vi "AnalysisTools.vi"(7 "Cali.Ref(Caller)":refnum<vi>) -> ()   [LabVIEW 2013]
uses:
  ProcessMethods/Binning/BinType.ctl
  <vilib>/Utility/miscctls.llb/LVRowAndColumnUnsignedTypeDef.ctl
  Files/Signal_Segment.ctl
  ControlDef/ProcessingMode.ctl
  <vilib>/Analysis/6fits.llb/General Linear Fit Algorithm.ctl
  <vilib>/Analysis/6fits.llb/Curve Fitting Criteria.ctl
  UI/Autoscale_Y_Multiple.vi
  ProcessMethods/Binning/SpectraBinning.vi
  ProcessMethods/MassResolutionCalc/FindMassResolution_Multiple.vi
  <vilib>/regexp/Match Regular Expression.xnode
  <vilib>/Analysis/NI_AALPro.lvlib
  <vilib>/Analysis/NI_AAL_SigProc.lvlib
  <vilib>/ptbypt/NI_PtbyPt.lvlib
panel:
  in  "Fullscale Y":bool
  in  "Y--":bool
  in  "Y++":bool
  in  "Res.":bool
  in  "Binning":bool
  in  "BinType":T1
  in  "BinWidth":dbl=1.0 min=0.001 max=32768.0 step=0.001 format="%.3f"
  in  "X++":bool
  in  "X--":bool
  in  "Fullscale X":bool
  in  "Reload":bool
  in  "Path":path
  out "Spectrum":cluster{dbl[], "Amplitudes":dbl[]}[](graph)
  in  "Tab Control":T2(tab)
  in  "Calibration Table":dbl[][](array[numeric]) caption="raw m/z"
  in  "Export_GraphData":bool
  in  "ApplyToFile":bool
  out "M/z curve fitting":cluster{"Y":dbl[], "Y":dbl[]}[](graph)
  in  "Calibration Coefficients":dbl[](array[numeric]) format="%.5f"
  out "R^2":dbl
  in  "Apply":bool
  in  "mzML Export":bool
  in  "ApplyToMainProgram":bool
  in  "AddSelection":bool
  in  "ExportPCA":bool
  in  "Multicolumn Listbox":i32[](listbox)
  in  "Search":bool
  in  "threshold":dbl format="%#_5p"
  in  "width":i32=3 min=3
  out "# found":i32
  in  "LoadMultiple...":bool
  in  "Reset":bool
  in  "ExportTable":bool
  in  "CopyPeakAreas":bool
  in  "CalcPeakAreas":bool
  in  "Selected Peak list":i32[](listbox)=[2]
  in  "Decode_regexp":string="Br2-Tyr_([-+]?[0-9]*[,\\.]?[0-9]+([eE][-+]?[0-9]+)?)%_([-+]?[0-9]*[,\\.]?[0-9]+([eE][-+]?[0-9]+)?)uJ_([-+]?[0-9]*[,\\.]?[0-9]+([eE][-+]?[0-9]+)?)us_([-+]?[0-9]*[,\\.]?[0-9]+([eE][-+]?[0-9]+)?).txt"
  in  "Decode_Filename?":bool
  in  "Accumulate":bool
  out "Accumulated Data":dbl[][](array[numeric])
  in  "Export+Proc":bool
  out "selected submatch":string
  in  "Submatch Selector":i32
  out "Referance Mass":string[][](table)=[["Compound", "", "mass", ""], ["Sexithiophone", "6T", "493.98", "s"], ["", "4T", "330.00", "s"], ["", "8T", "657.96", "w"], ["NPM", "M+", "297", "s"], ["", "", "217", "w"], ["CHCA", "M+", "189.04", "s"], ["DHB", "M+", "154.03", "s"], ["Rifampcin", "", "", ""], ["Tantalum", "", "", ""], ["Cu", "63", "", ""], ["", "65", "", ""], ["Mo", "", "", ""]]
  in  "m/z":dbl
  in  "time":dbl
  in  "Add to":bool
  out "Original m/z":dbl
  in  "Calc Calibration":bool
  in  "Quit":bool
  # "raw m/z"
  # "time"
  # "cali. m/z"
  # "delta m/z"
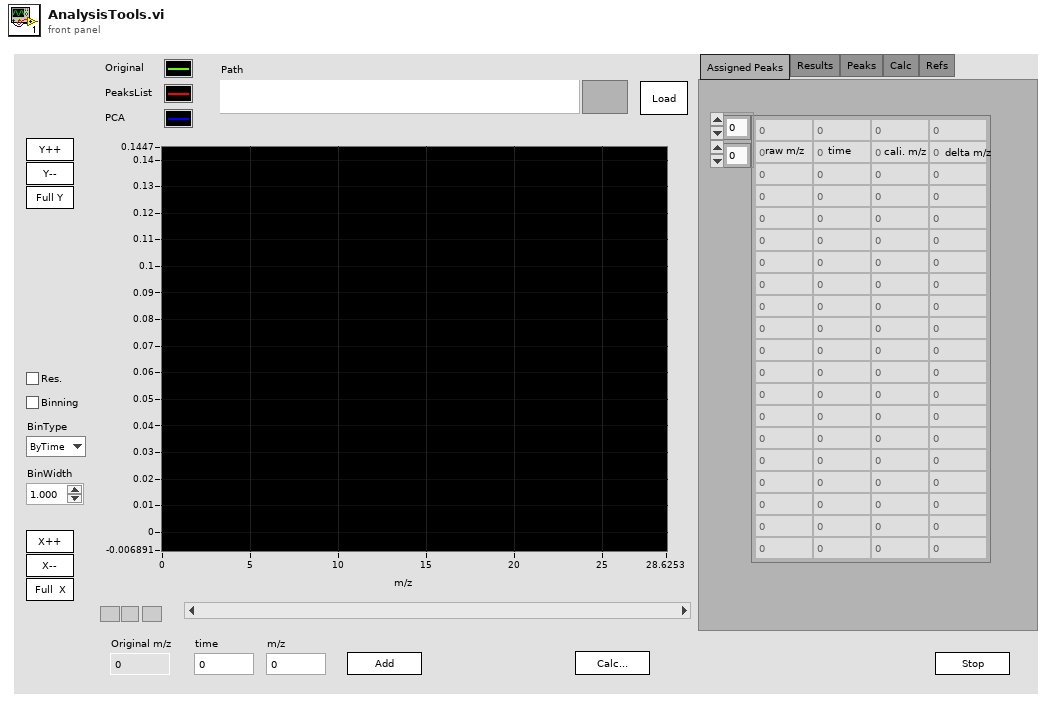
[diagram p1: front panel]
types:
  T1 = typedef "BinType.ctl" = enum16{"ByTime", "ByScreen", "ByMass", "ToUnitMass"}
  T2 = enum32{"Assigned Peaks", "Results", "Peaks", "Calc", "Refs"}
  T3 = typedef "LVRowAndColumnUnsignedTypeDef.ctl" = cluster{"Row":u32, "Column":u32}
  T4 = cluster{"Plot.Bar Plot Style":u8, "Plot.Plot Color":u32, "Plot.Line Style":u8, "Plot.Plot Interpolation":u8, "Plot.Plot Name":string, "Plot.Point Style":u8, "Plot.Visible":bool}[]
  T5 = typedef "Signal_Segment.ctl" = cluster{"SampleRate":dbl, "TrigDelay":dbl, "SpecLength":dbl, "DAQ_Range":dbl, "Average#":i32, "Position":dbl[], "Spectrum":sgl[], "Calibr.":dbl[], "Pressure":dbl, "Desp_LaserEnergy":dbl, "PI_LaserEnergy":dbl, "Voltages Table":sgl[][], "ProcMode":T6, "Threshold":dbl, "Comment":string, "TickCount":dbl, "Time Stamp":timestamp}
  T6 = typedef "ProcessingMode.ctl" = enum16{"None", "Drop by Threshold", "TDC Simulate", "SetFilter"}
  T7 = cluster{"Spectrum":T5, "Peaks Table":dbl[][], "BinnedSpec":cluster{"m/z":dbl[], "Intensity":dbl[]}, "PeaksList":cluster{"m/z":dbl[], "Intensity":dbl[]}, "PCA":cluster{"m/z":dbl[], "Intensity":dbl[]}, "m/z":dbl[], "InitialCali.":dbl[], "Filename":string, "AccumulatedPeakAreas":cluster{"Labels":string[], "Areas":dbl[][], "Areas^2":dbl[][], "n":i32[]}, "app vi reference":refnum<vi>}
  T8 = cluster{"Labels":string[], "Areas":dbl[][], "Areas^2":dbl[][], "n":i32[]}
  T9 = typedef "LVPoint32TypeDef.ctl" = cluster{"Horizontal":i32, "Vertical":i32}
  T10 = typedef "NI_AALPro.lvlib/Curve Fitting Criteria.ctl" = u16
  T11 = typedef "NI_AALPro.lvlib/General Linear Fit Algorithm.ctl" = u16
  T12 = cluster{"Calibration Table":dbl[], "Calibration Table":dbl[]}
  T13 = cluster{"Calibration Table":dbl[], "Calibration Table":dbl[]}[]
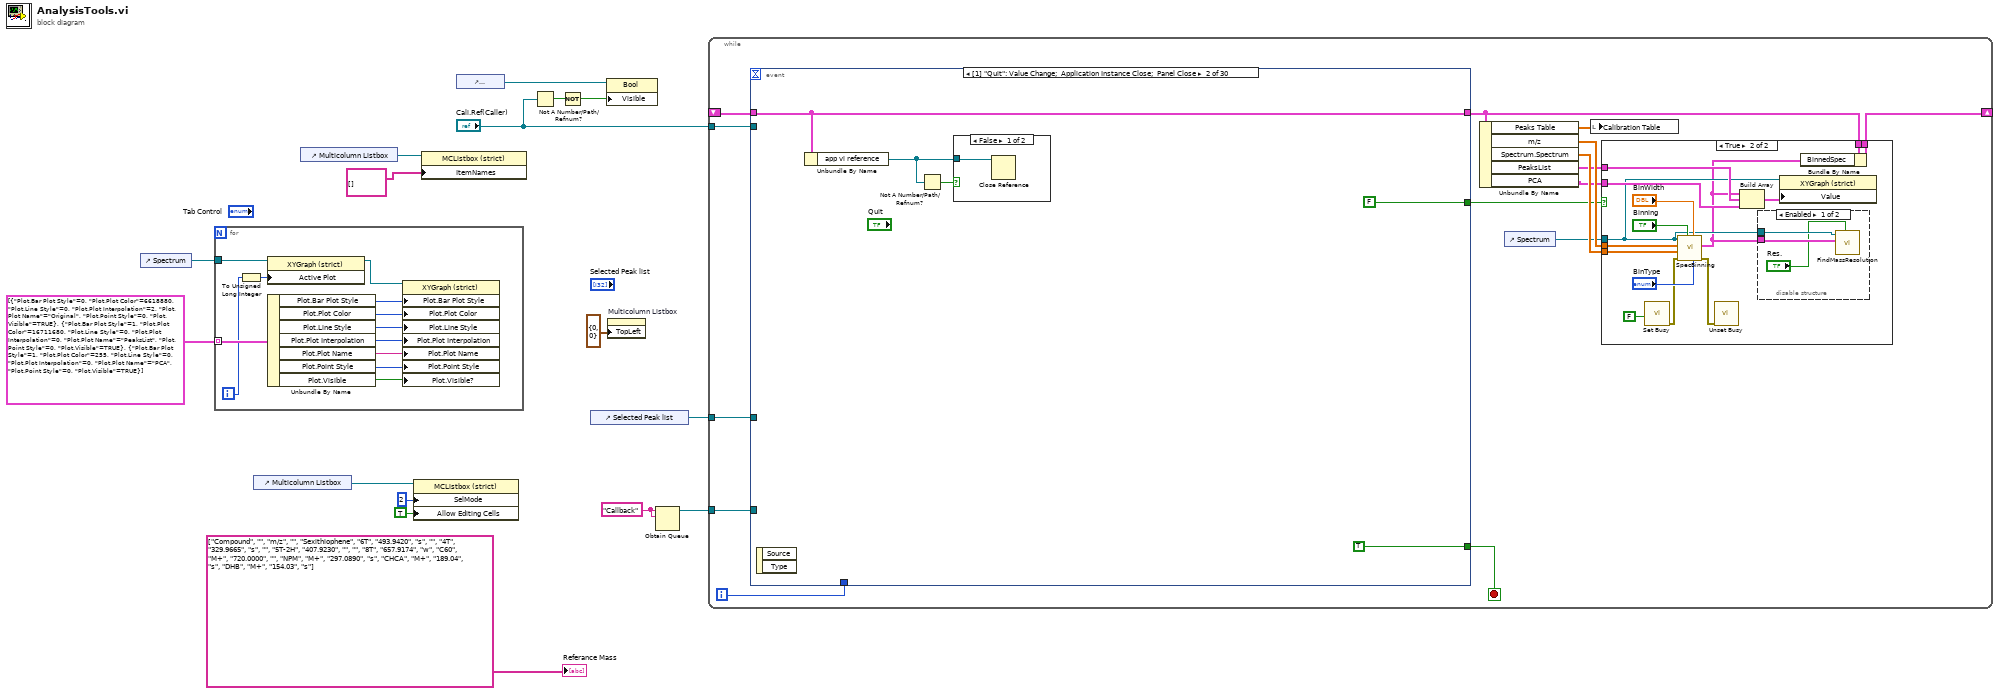
[diagram p0: block diagram]
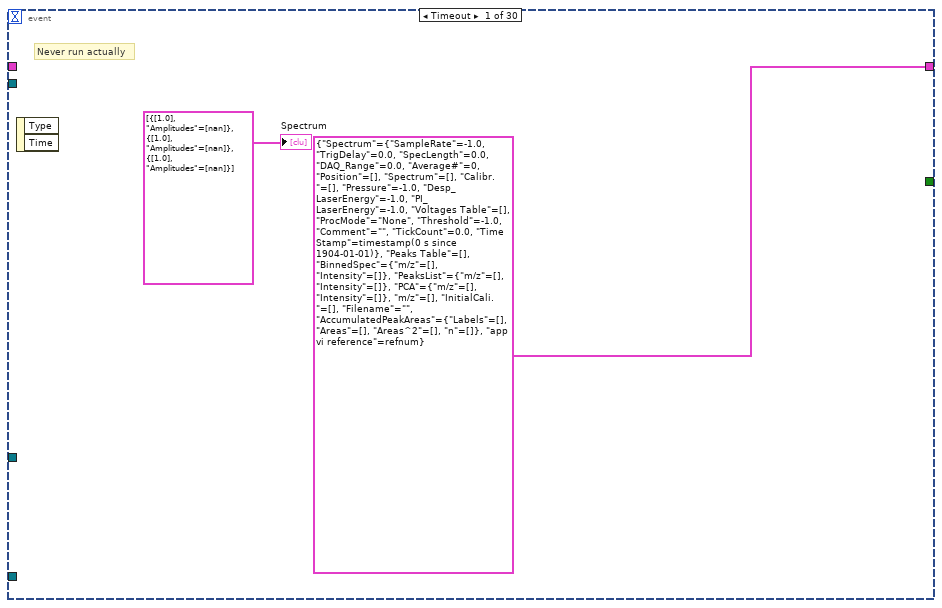
[diagram p4: hidden frame]
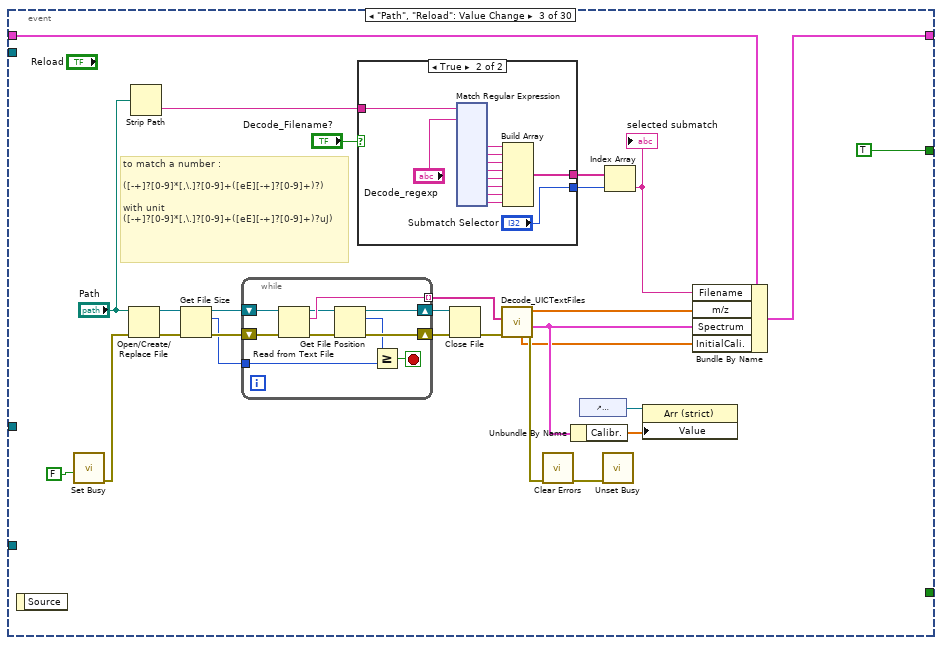
[diagram p6: hidden frame]
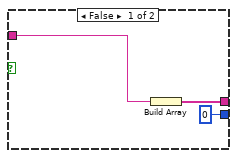
[diagram p7: hidden frame]
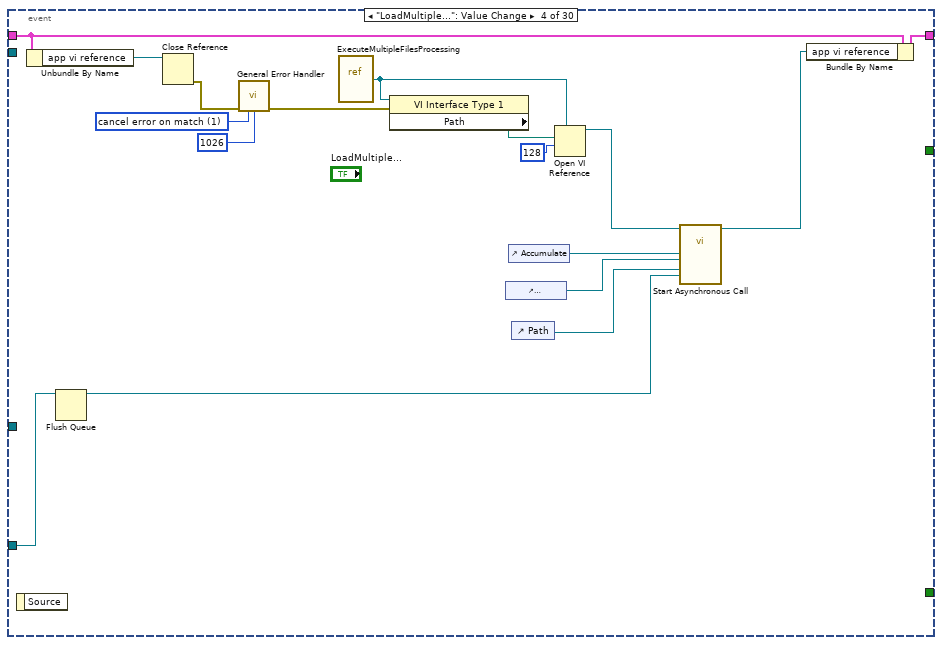
[diagram p8: hidden frame]
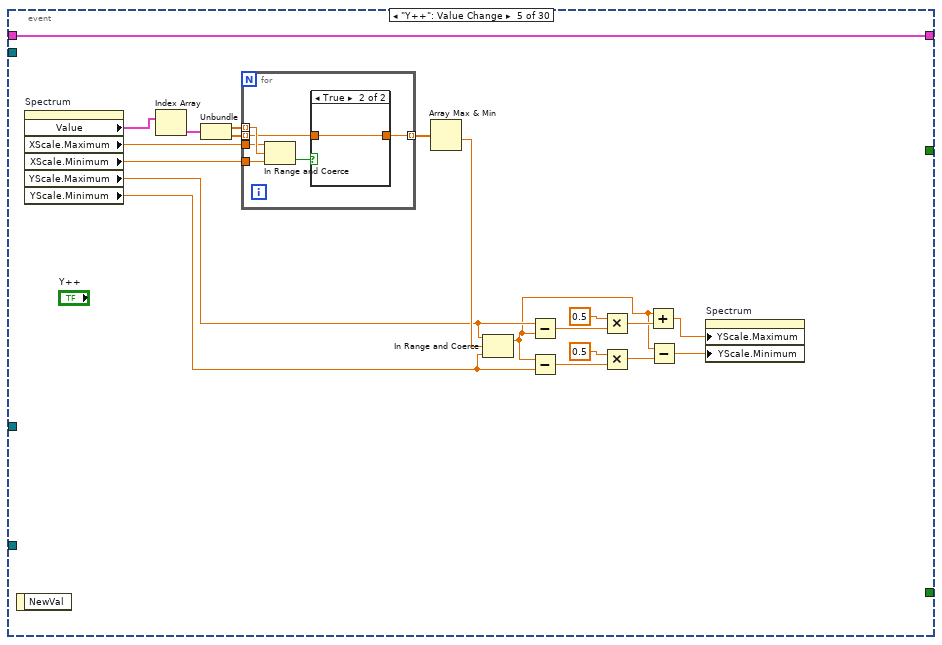
[diagram p9: hidden frame]
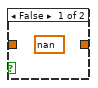
[diagram p10: hidden frame]
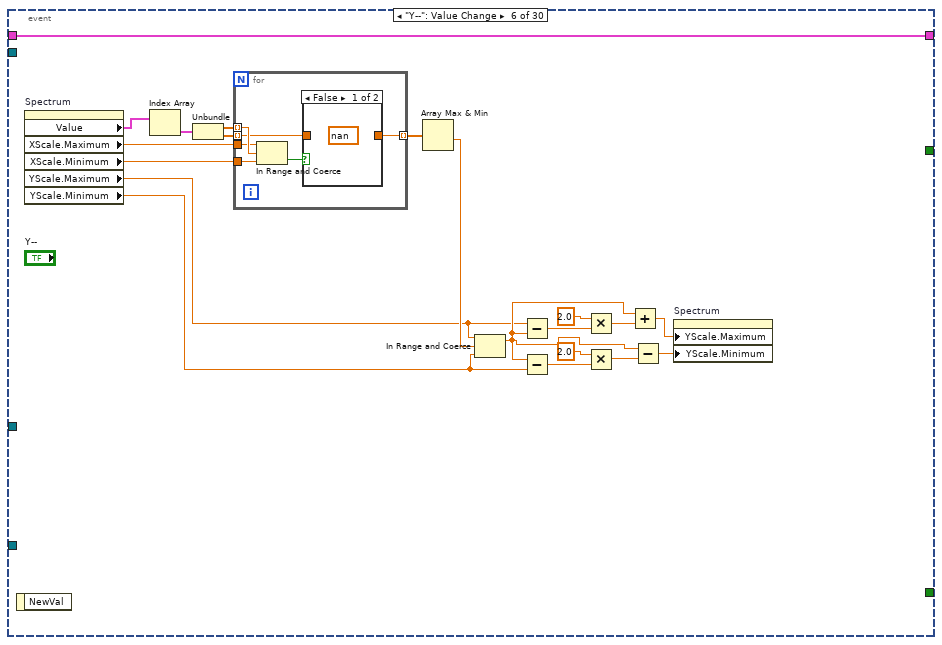
[diagram p11: hidden frame]
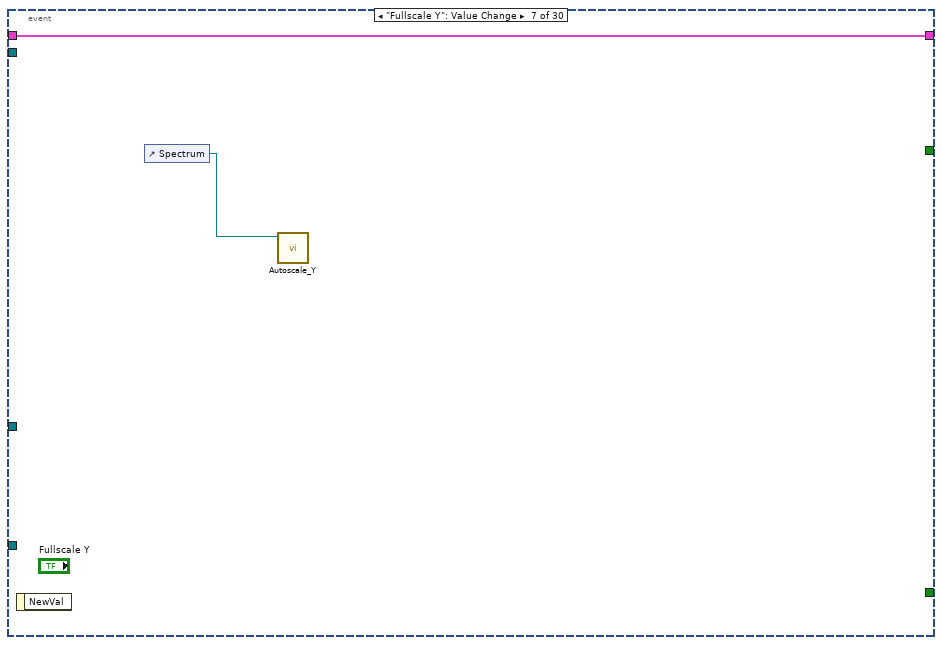
[diagram p13: hidden frame]
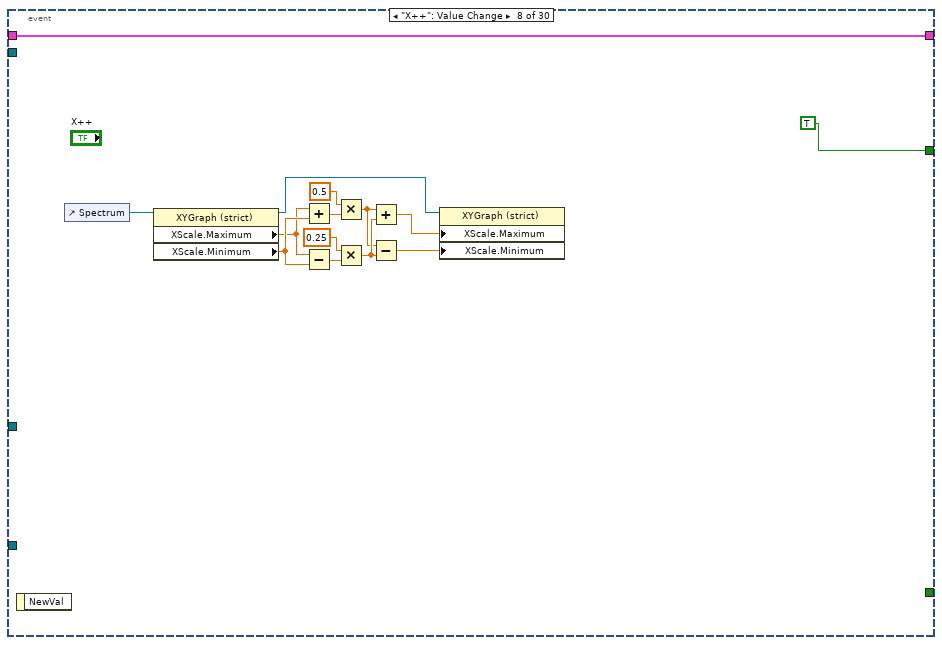
[diagram p14: hidden frame]
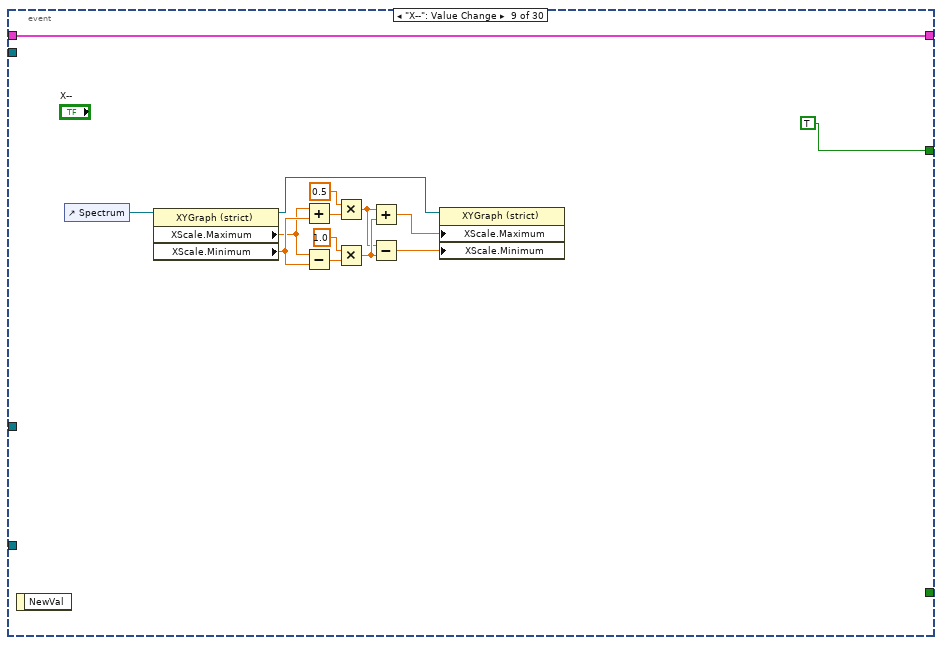
[diagram p15: hidden frame]
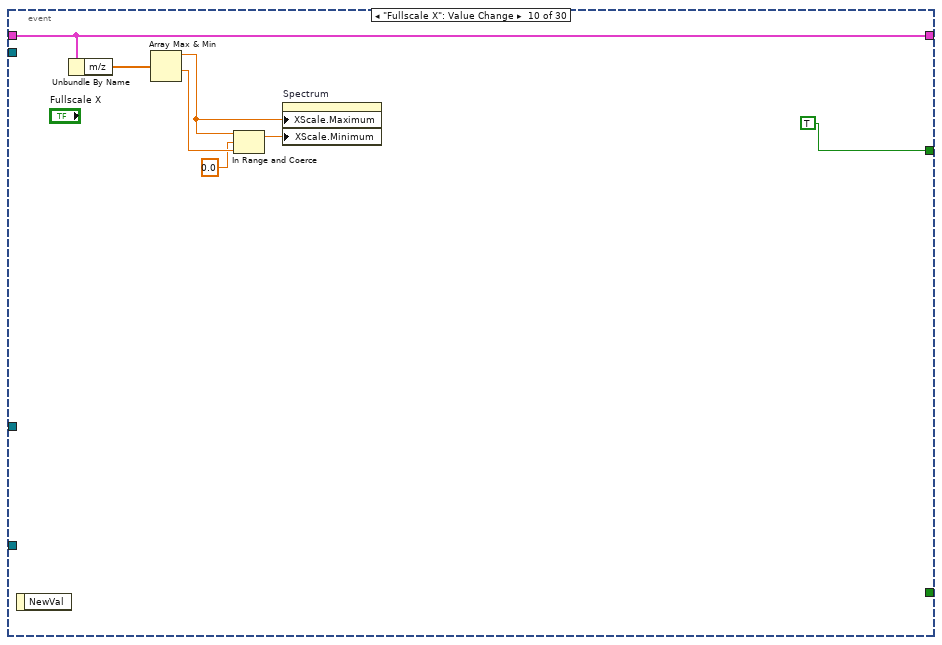
[diagram p16: hidden frame]
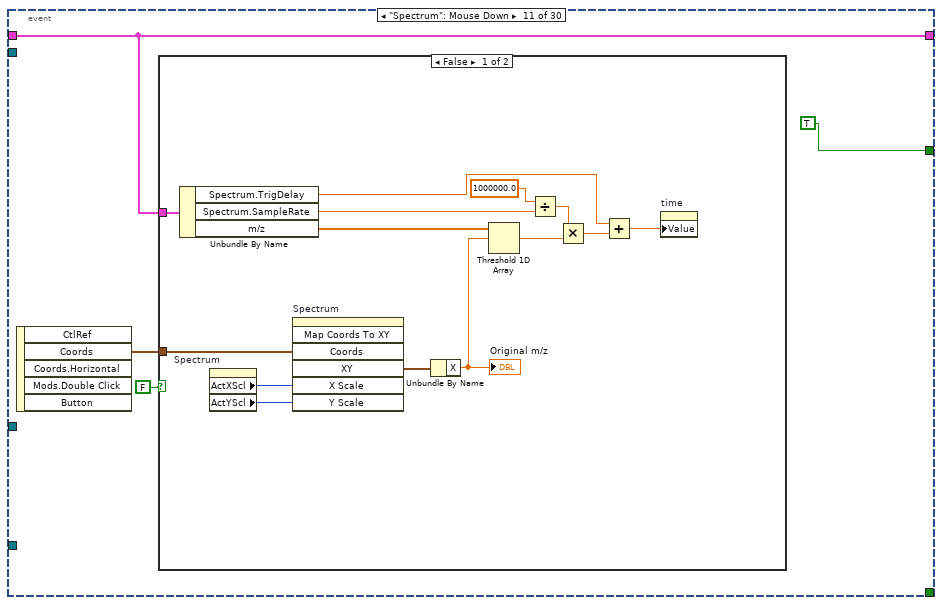
[diagram p17: hidden frame]
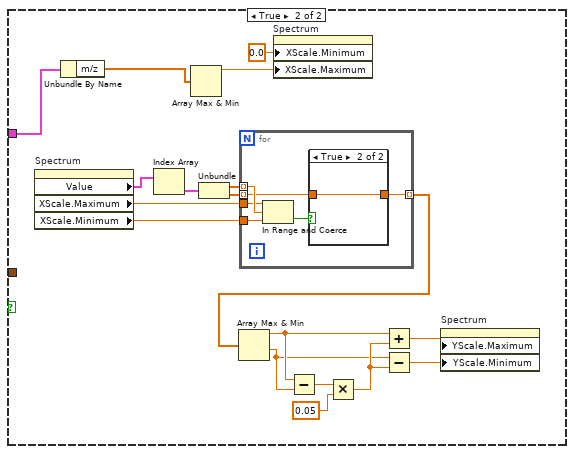
[diagram p18: hidden frame]
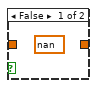
[diagram p19: hidden frame]
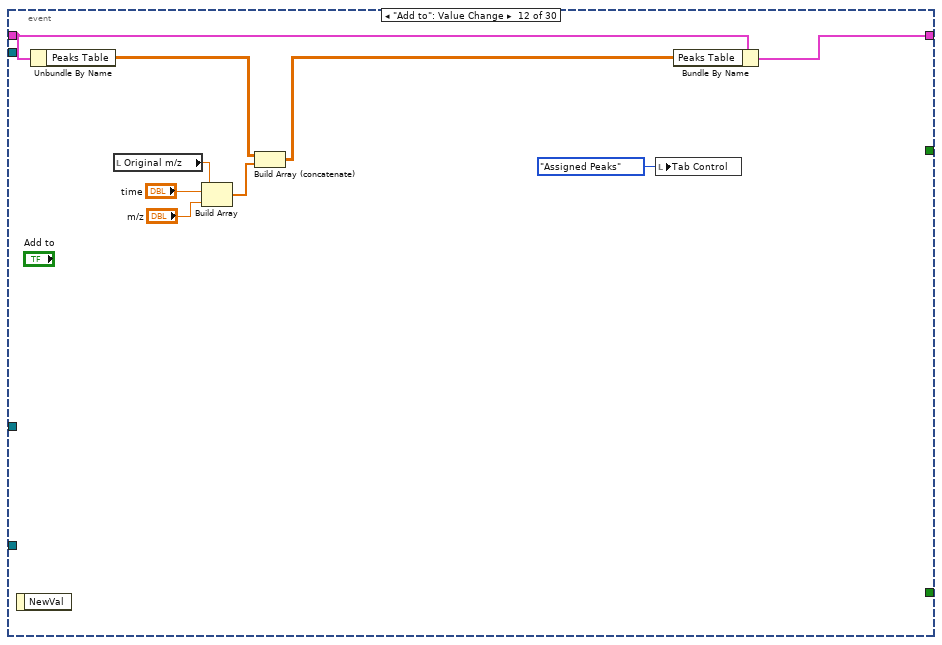
[diagram p20: hidden frame]
diagram:
  w9 = "Callback" ("name (unnamed)")
  n1 = control-ref of="Spectrum"() -> (w14:refnum<vi>)
  n2 = for {
    tunnel: w14 -> [w28]
    tunnel: T4 [{"Plot.Bar Plot Style"=0, "Plot.Plot Color"=6618880, "Plot.Line Style"=0, "Plot.Plot Interpolation"=2, "Plot.Plot Name"="Original", "Plot.Point Style"=0, "Plot.Visible"=TRUE}, {"Plot.Bar Plot Style"=1, "Plot.Plot Color"=16711680, "Plot.Line Style"=0, "Plot.Plot Interpolation"=0, "Plot.Plot Name"="PeaksList", "Plot.Point Style"=0, "Plot.Visible"=TRUE}, {"Plot.Bar Plot Style"=1, "Plot.Plot Color"=255, "Plot.Line Style"=0, "Plot.Plot Interpolation"=0, "Plot.Plot Name"="PCA", "Plot.Point Style"=0, "Plot.Visible"=TRUE}] -> [w26] mode=indexing
    i -> [w18]
    n3 = To Unsigned Long Integer(number=w18) -> (unsigned 32bit integer=w17:u32)
    n4 = property class="XYGraph (strict)"(reference=w28, "Active Plot"=w17) -> (reference out=w27:refnum<vi>)  [unwired: 1 in, 1 out]
    n5 = Unbundle By Name(w26) -> ("Plot.Bar Plot Style"=w21:u8, "Plot.Plot Color"=w22:u32, "Plot.Line Style"=w19:u8, "Plot.Plot Interpolation"=w20:u8, "Plot.Plot Name"=w23:string, "Plot.Point Style"=w24:u8, "Plot.Visible"=w25:bool)
    n6 = property class="XYGraph (strict)"(reference=w27, "Plot.Bar Plot Style"=w21, "Plot.Plot Color"=w22, "Plot.Line Style"=w19, "Plot.Plot Interpolation"=w20, "Plot.Plot Name"=w23, "Plot.Point Style"=w24, "Plot.Visible?"=w25) -> ()  [unwired: 1 in, 2 out]
  }
  n7 = control-ref of="Multicolumn Listbox"() -> (w13:refnum<vi>)
  n8 = control-ref of="Multicolumn Listbox"() -> (w2:refnum<vi>)
  n9 = property class="MCListbox (strict)"(reference=w13, "SelMode"=2 ("Selection Mode"), "Allow Editing Cells"=TRUE) -> ()  [unwired: 1 in, 2 out]
  n10 = property class="MCListbox (strict)"(reference=w2, "ItemNames"=string[][] [] ("Item Names")) -> ()  [unwired: 1 in, 2 out]
  n11 = control-ref of="ApplyToMainProgram"() -> (w4:refnum<vi>)
  n12 = Not A Number/Path/Refnum?(number/path/refnum="Cali.Ref(Caller)") -> (NaN/Path/Refnum?=w6:bool)
  n13 = Not(x=w6) -> (.not. x?=w5:bool)
  n14 = control-ref of="Selected Peak list"() -> (w7:refnum<vi>)
  n15 = property class="Bool"(reference=w4, "Visible"=w5) -> ()  [unwired: 1 in, 2 out]
  n16 = property on="Multicolumn Listbox" class="MCListbox (strict)"("TopLeft"=T3 {"Row"=0, "Column"=0} ("Top Left Visible Cell")) -> ()  [unwired: 2 in, 2 out]
  n17 = Obtain Queue(name (unnamed)=w9, element data type=w9) -> (queue out=w8:refnum<queue>)  [unwired: 3 in, 2 out]
  n18 = while {
    shift-right: [w36] -> _
    shift-left: _ -> [w43]
    tunnel: w8 -> [w31]
    tunnel: w7 -> [w30]
    tunnel: "Cali.Ref(Caller)" -> [w29]
    i -> [w32]
    stop <- w41 stop-if-true
    n19 = event shown="[1] \"Quit\": Value Change;  Application Instance Close;  Panel Close" {
      selector: _ -> [_ _ _ _ _ _ _ _ _ _ _ _ _ _ _ _ _ _ _ _ _ _ _ _ _ _ _ _ _ _]
      dyn-events: _ -> [_ _ _ _ _ _ _ _ _ _ _ _ _ _ _ _ _ _ _ _ _ _ _ _ _ _ _ _ _ _]
      timeout: _ -> [_ _ _ _ _ _ _ _ _ _ _ _ _ _ _ _ _ _ _ _ _ _ _ _ _ _ _ _ _ _]
      tunnel: [T7 {"Spectrum"={"SampleRate"=-1.0, "TrigDelay"=0.0, "SpecLength"=0.0, "DAQ_Range"=0.0, "Average#"=0, "Position"=[], "Spectrum"=[], "Calibr."=[], "Pressure"=-1.0, "Desp_LaserEnergy"=-1.0, "PI_LaserEnergy"=-1.0, "Voltages Table"=[], "ProcMode"=enum."None", "Threshold"=-1.0, "Comment"="", "TickCount"=0.0, "Time Stamp"=timestamp(0 s since 1904-01-01)}, "Peaks Table"=[], "BinnedSpec"={"m/z"=[], "Intensity"=[]}, "PeaksList"={"m/z"=[], "Intensity"=[]}, "PCA"={"m/z"=[], "Intensity"=[]}, "m/z"=[], "InitialCali."=[], "Filename"="", "AccumulatedPeakAreas"={"Labels"=[], "Areas"=[], "Areas^2"=[], "n"=[]}, "app vi reference"=refnum} w67 w97 w253 w279 w306 w318 w332 w346 w353 w356 w403 w407 w448 w483 w503 w534 w537 w547 w665 w695 w738 w742 w747 w872 w893 w915 w933 w966 w1007] -> w37
      tunnel: w43 -> [_ w67 w96 w251 w279 w306 w318 w332 w346 w353 w356 w404 w407 w440 w482 w503 w534 w537 w547 w666 w696 w738 w743 w747 w872 w893 w915 w933 w967 w1008]
      tunnel: [_ TRUE _ _ _ _ _ _ _ _ _ _ _ _ _ _ _ _ _ _ _ _ _ _ _ _ _ _ _ _] -> w41
      tunnel: [_ FALSE TRUE _ _ _ _ TRUE TRUE TRUE TRUE _ TRUE TRUE TRUE TRUE _ _ _ TRUE _ _ _ _ _ _ _ _ _ _] -> w38
      tunnel: w32 -> [_ _ _ _ _ _ _ _ _ _ _ _ _ _ _ _ _ _ _ _ _ _ _ _ _ _ _ _ _ _]
      tunnel: w31 -> [_ _ _ w255 _ _ _ _ _ _ _ _ _ _ _ _ _ _ _ _ _ _ _ _ _ _ _ _ w964 _]
      tunnel: w30 -> [_ _ _ _ _ _ _ _ _ _ _ _ _ _ _ _ _ _ _ _ _ _ _ _ _ _ _ _ w963 _]
      tunnel: w29 -> [_ _ _ _ _ _ _ _ _ _ _ _ _ _ _ _ _ w535 _ _ _ _ _ _ _ _ _ _ _ _]
      event Timeout {
        # "Never run actually"
        n20 = event-data() -> ()  [unwired: 1 in, 2 out]
        "Spectrum" <- cluster{dbl[], "Amplitudes":dbl[]}[] [{[1.0], "Amplitudes"=[nan]}, {[1.0], "Amplitudes"=[nan]}, {[1.0], "Amplitudes"=[nan]}]
      }
      event "Quit": Value Change; Application Instance Close; Panel Close {
        n21 = event-data() -> ()  [unwired: 1 in, 2 out]
        n22 = Unbundle By Name(w67) -> ("app vi reference"=w65:refnum<vi>)
        n23 = Not A Number/Path/Refnum?(number/path/refnum=w65) -> (NaN/Path/Refnum?=w66:bool)
        n24 = case shown="False" w66 {
          tunnel: w65 -> [w70 _]
          frame False {
            n25 = Close Reference(reference=w70) -> ()  [unwired: 1 in, 1 out]
          }
          frame True {
          }
        }
      }
      event "Path", "Reload": Value Change {
        # "to match a number :\n\n([-+]?[0-9]*[,\\.]?[0-9]+([eE][-+]?[0-9]+)?)\n\nwith unit \n([-+]?[0-9]*[,\\.]?[0-9]+([eE][-+]?[0-9]+)?uJ)"
        n26 = event-data() -> ()  [unwired: 1 in, 1 out]
        n27 = call <vilib>:"Set Busy.vi"("disable click? (T)"=FALSE) -> ("error out"=w86:errorcluster)  [unwired: 9 in, 1 out]
        n28 = Open/Create/Replace File(file path (use dialog)="Path", error in=w86) -> (refnum out=w94:refnum<file>, error out=w95:errorcluster)  [unwired: 4 in, 1 out]
        n29 = Strip Path(path="Path") -> (name=w75:string)  [unwired: 1 out]
        n30 = Get File Size(file=w94, error in=w95) -> (refnum out=w92:refnum<file>, size (in bytes)=w90:i64, 0:w93:errorcluster)
        n31 = while {
          shift-right: [w241] -> w80
          shift-left: w92 -> [w245]
          shift-right: [w240] -> w79
          shift-left: w93 -> [w244]
          tunnel: [w243] -> w91 mode=indexing
          tunnel: w90 -> [w237]
          stop <- w236 stop-if-true
          n32 = Read from Text File(file (use dialog)=w245, error in=w244) -> (refnum out=w242:refnum<file>, text=w243:string, error out=w239:errorcluster)  [unwired: 2 in, 1 out]
          n33 = Get File Position(4:w239, 7:w242) -> (0:w240:errorcluster, 2:w238:i64, 3:w241:refnum<file>)
          n34 = Greater Or Equal?(x=w238, y=w237) -> (x >= y?=w236:bool)
        }
        n35 = case shown="True" "Decode_Filename?" {
          tunnel: w75 -> [w99 w111]
          tunnel: [w100 w102] -> w72
          tunnel: [0 ("Submatch Selector") "Submatch Selector"] -> w71
          frame False {
            n36 = Build Array(w99) -> (w100:string[])
          }
          frame True {
            n37 = xnode "Match Regular Expression"("input string"=w111, "regular expression"="Decode_regexp") -> ("submatch 1"=w110:string, "submatch 2"=w109:string, "submatch 3"=w108:string, "submatch 4"=w107:string, "submatch 5"=w106:string, "submatch 6"=w105:string, "submatch 7"=w104:string, "submatch 8"=w103:string)  [unwired: 4 in, 5 out]
            n38 = Build Array(w110, w109, w108, w107, w106, w105, w104, w103) -> (w102:string[])
          }
        }
        n39 = Close File(refnum=w80, error in=w79) -> (error out=w78:errorcluster)  [unwired: 1 out]
        n40 = call "Decode_UICTextFiles.vi"("error in"=w78, "Text Array"=w91) -> ("error out"=w89:errorcluster, "Spectrum"=w83:T5, "m/z list"=w84:dbl[], "InitialCali."=w77:dbl[])  [unwired: 5 in, 1 out]
        n41 = call <vilib>:"Clear Errors.vi"("error in (no error)"=w89) -> ("error out"=w85:errorcluster)  [unwired: 6 in]
        n42 = Unbundle By Name(w83) -> ("Calibr."=w81:dbl[])
        n43 = control-ref of="Calibration Coefficients"() -> (w82:refnum<vi>)
        n44 = call <vilib>:"Unset Busy.vi"("error in (no error)"=w85) -> ()  [unwired: 10 in, 1 out]
        n45 = Index Array(array=w72, index=w71) -> (element=w73:string)
        "selected submatch" <- w73
        n46 = property class="Arr (strict)"(reference=w82, "Value"=w81) -> ()  [unwired: 1 in, 2 out]
        n47 = Bundle By Name(cluster=w96, "Filename"=w73, "m/z"=w84, "Spectrum"=w83, "InitialCali."=w77) -> (w97:T7)
      }
      event "LoadMultiple...": Value Change {
        w247 = 1 items=["no exception", "cancel error on match", "set error on match"] ("[exception action] (none:0)")
        n48 = event-data() -> ()  [unwired: 1 in, 1 out]
        n49 = Unbundle By Name(w251) -> ("app vi reference"=w250:refnum<vi>)
        n50 = Flush Queue(queue=w255) -> (queue out=w254:refnum<queue>)  [unwired: 1 in, 2 out]
        n51 = Close Reference(reference=w250) -> (error out=w249:errorcluster)  [unwired: 1 in]
        n52 = call <vilib>:"General Error Handler.vi"("error in (no error)"=w249, "[exception action] (none:0)"=w247, "[exception code]"=1026) -> ("error out"=w248:errorcluster)  [unwired: 8 in, 4 out]
        n53 = vi-ref "ExecuteMultipleFilesProcessing.vi"() -> (w262:refnum<vi>)
        n54 = property class="VI Interface Type 1"(reference=w262, error in=w248) -> ("Path"=w261:path)  [unwired: 2 out]
        n55 = control-ref of="CalcPeakAreas"() -> (w257:refnum<vi>)
        n56 = control-ref of="Accumulate"() -> (w258:refnum<vi>)
        n57 = control-ref of="Path"() -> (w256:refnum<vi>)
        n58 = Open VI Reference(type specifier VI Refnum (for type only)=w262, vi path=w261, options=128) -> (vi reference=w259:refnum<vi>)  [unwired: 3 in, 1 out]
        n59 = call-by-ref "Start Asynchronous Call"(reference=w259, "Callback queue in"=w254, "Path"=w256, "CalcPeakAreas"=w257, "Accumulate"=w258) -> (reference out=w252:refnum<vi>)  [unwired: 9 in, 1 out]
        n60 = Bundle By Name(cluster=w251, "app vi reference"=w252) -> (w253:T7)
      }
      event "Y++": Value Change {
        n61 = event-data() -> ()  [unwired: 1 in, 1 out]
        n62 = property on="Spectrum" class="XYGraph (strict)"() -> ("Value"=w268:cluster{dbl[], "Amplitudes":dbl[]}[], "XScale.Maximum"=w276:dbl, "XScale.Minimum"=w275:dbl, "YScale.Maximum"=w265:dbl, "YScale.Minimum"=w264:dbl)  [unwired: 2 in, 2 out]
        n63 = Index Array(array=w268) -> (element=w267:cluster{dbl[], "Amplitudes":dbl[]})  [unwired: 1 in]
        n64 = Unbundle(w267) -> (w278:dbl[], "Amplitudes"=w277:dbl[])
        n65 = for {
          tunnel: w277 -> [w284] mode=indexing
          tunnel: w278 -> [w288] mode=indexing
          tunnel: w275 -> [w287]
          tunnel: w276 -> [w286]
          tunnel: [w283] -> w274 mode=indexing
          n66 = In Range and Coerce(upper limit=w286, x=w288, lower limit=w287) -> (In Range?=w285:bool)  [unwired: 1 out]
          n67 = case shown="True" w285 {
            tunnel: w284 -> [_ w289]
            tunnel: [_ w289] -> w283
            frame False {
              (unwired) nan
            }
            frame True {
            }
          }
        }
        n68 = Array Max & Min(array=w274) -> (min value=w266:dbl)  [unwired: 3 out]
        n69 = In Range and Coerce(upper limit=w265, x=w266, lower limit=w264) -> (coerced(x)=w263:dbl)  [unwired: 1 out]
        n70 = Subtract(x=w265, y=w263) -> (x-y=w273:dbl)
        n71 = Subtract(x=w263, y=w264) -> (x-y=w271:dbl)
        n72 = Multiply(x=0.5, y=w273) -> (x*y=w281:dbl)
        n73 = Multiply(x=0.5, y=w271) -> (x*y=w270:dbl)
        n74 = Add(x=w263, y=w281) -> (x+y=w280:dbl)
        n75 = Subtract(x=w263, y=w270) -> (x-y=w269:dbl)
        n76 = property on="Spectrum" class="XYGraph (strict)"("YScale.Maximum"=w280, "YScale.Minimum"=w269) -> ()  [unwired: 2 in, 2 out]
      }
      event "Y--": Value Change {
        n77 = event-data() -> ()  [unwired: 1 in, 1 out]
        n78 = property on="Spectrum" class="XYGraph (strict)"() -> ("Value"=w305:cluster{dbl[], "Amplitudes":dbl[]}[], "XScale.Maximum"=w302:dbl, "XScale.Minimum"=w301:dbl, "YScale.Maximum"=w291:dbl, "YScale.Minimum"=w290:dbl)  [unwired: 2 in, 2 out]
        n79 = Index Array(array=w305) -> (element=w294:cluster{dbl[], "Amplitudes":dbl[]})  [unwired: 1 in]
        n80 = Unbundle(w294) -> (w304:dbl[], "Amplitudes"=w303:dbl[])
        n81 = for {
          tunnel: w303 -> [w311] mode=indexing
          tunnel: w304 -> [w315] mode=indexing
          tunnel: w301 -> [w314]
          tunnel: w302 -> [w313]
          tunnel: [w310] -> w300 mode=indexing
          n82 = In Range and Coerce(upper limit=w313, x=w315, lower limit=w314) -> (In Range?=w312:bool)  [unwired: 1 out]
          n83 = case shown="False" w312 {
            tunnel: w311 -> [_ w316]
            tunnel: [_ w316] -> w310
            frame False {
              (unwired) nan
            }
            frame True {
            }
          }
        }
        n84 = Array Max & Min(array=w300) -> (min value=w292:dbl)  [unwired: 3 out]
        n85 = In Range and Coerce(upper limit=w291, x=w292, lower limit=w290) -> (coerced(x)=w293:dbl)  [unwired: 1 out]
        n86 = Subtract(x=w291, y=w293) -> (x-y=w299:dbl)
        n87 = Subtract(x=w293, y=w290) -> (x-y=w297:dbl)
        n88 = Multiply(x=2.0, y=w299) -> (x*y=w308:dbl)
        n89 = Multiply(x=2.0, y=w297) -> (x*y=w296:dbl)
        n90 = Add(x=w293, y=w308) -> (x+y=w307:dbl)
        n91 = Subtract(x=w293, y=w296) -> (x-y=w295:dbl)
        n92 = property on="Spectrum" class="XYGraph (strict)"("YScale.Maximum"=w307, "YScale.Minimum"=w295) -> ()  [unwired: 2 in, 2 out]
      }
      event "Fullscale Y": Value Change {
        n93 = event-data() -> ()  [unwired: 1 in, 1 out]
        n94 = control-ref of="Spectrum"() -> (w317:refnum<vi>)
        n95 = call-poly "Autoscale_Y.vi"("GraphRef"=w317) -> ()  [unwired: 11 in]
      }
      event "X++": Value Change {
        n96 = event-data() -> ()  [unwired: 1 in, 1 out]
        n97 = control-ref of="Spectrum"() -> (w321:refnum<vi>)
        n98 = property on="Property Node" class="XYGraph (strict)"(reference=w321) -> (reference out=w320:refnum<vi>, "XScale.Maximum"=w322:dbl, "XScale.Minimum"=w323:dbl)  [unwired: 1 in, 1 out]
        n99 = Add(x=w322, y=w323) -> (x+y=w324:dbl)
        n100 = Subtract(x=w322, y=w323) -> (x-y=w327:dbl)
        n101 = Multiply(x=0.5, y=w324) -> (x*y=w328:dbl)
        n102 = Multiply(x=0.25, y=w327) -> (x*y=w329:dbl)
        n103 = Add(x=w328, y=w329) -> (x+y=w330:dbl)
        n104 = Subtract(x=w328, y=w329) -> (x-y=w331:dbl)
        n105 = property on="Property Node" class="XYGraph (strict)"(reference=w320, "XScale.Maximum"=w330, "XScale.Minimum"=w331) -> ()  [unwired: 1 in, 2 out]
      }
      event "X--": Value Change {
        n106 = event-data() -> ()  [unwired: 1 in, 1 out]
        n107 = control-ref of="Spectrum"() -> (w335:refnum<vi>)
        n108 = property on="Property Node" class="XYGraph (strict)"(reference=w335) -> (reference out=w334:refnum<vi>, "XScale.Maximum"=w336:dbl, "XScale.Minimum"=w337:dbl)  [unwired: 1 in, 1 out]
        n109 = Add(x=w336, y=w337) -> (x+y=w338:dbl)
        n110 = Subtract(x=w336, y=w337) -> (x-y=w341:dbl)
        n111 = Multiply(x=0.5, y=w338) -> (x*y=w342:dbl)
        n112 = Multiply(x=1.0, y=w341) -> (x*y=w343:dbl)
        n113 = Add(x=w342, y=w343) -> (x+y=w344:dbl)
        n114 = Subtract(x=w342, y=w343) -> (x-y=w345:dbl)
        n115 = property on="Property Node" class="XYGraph (strict)"(reference=w334, "XScale.Maximum"=w344, "XScale.Minimum"=w345) -> ()  [unwired: 1 in, 2 out]
      }
      event "Fullscale X": Value Change {
        n116 = event-data() -> ()  [unwired: 1 in, 1 out]
        n117 = Unbundle By Name(w353) -> ("m/z"=w347:dbl[])
        n118 = Array Max & Min(array=w347) -> (max value=w348:dbl, min value=w351:dbl)  [unwired: 2 out]
        n119 = In Range and Coerce(upper limit=w348, x=0.0 ("X Scale.Range:Minimum"), lower limit=w351) -> (coerced(x)=w349:dbl)  [unwired: 1 out]
        n120 = property on="Spectrum" class="XYGraph (strict)"("XScale.Maximum"=w348, "XScale.Minimum"=w349) -> ()  [unwired: 2 in, 2 out]
      }
      event "Spectrum": Mouse Down {
        n121 = event-data() -> ("Coords"=w357:T9)  [unwired: 1 in, 4 out]
        n122 = case shown="False" FALSE {
          tunnel: w357 -> [w371 _]
          tunnel: w356 -> [w367 w387]
          frame False {
            n123 = Unbundle By Name(w367) -> ("Spectrum.TrigDelay"=w359:dbl, "Spectrum.SampleRate"=w358:dbl, "m/z"=w361:dbl[])
            n124 = property on="Spectrum" class="XYGraph (strict)"() -> ("ActXScl"=w370:i32, "ActYScl"=w369:i32)  [unwired: 2 in, 2 out]
            n125 = invoke on="Spectrum" class="XYGraph (strict)" method="Map Coords To XY"("Coords"=w371, "X Scale"=w370, "Y Scale"=w369) -> ("XY"=w368:cluster{"X":dbl, "Y":dbl})  [unwired: 4 in, 6 out]
            n126 = Unbundle By Name(w368) -> ("X"=w362:dbl)
            "Original m/z" <- w362
            n127 = Threshold 1D Array(2:w362, 3:w361) -> (0:w364:dbl)  [unwired: 1 in]
            n128 = Divide(x=1000000.0, y=w358) -> (x/y=w365:dbl)
            n129 = Multiply(x=w365, y=w364) -> (x*y=w363:dbl)
            n130 = Add(x=w359, y=w363) -> (x+y=w360:dbl)
            n131 = property on="time" class="DigNum (strict)"("Value"=w360) -> ()  [unwired: 2 in, 2 out]
          }
          frame True {
            n132 = property on="Spectrum" class="XYGraph (strict)"() -> ("Value"=w386:cluster{dbl[], "Amplitudes":dbl[]}[], "XScale.Maximum"=w383:dbl, "XScale.Minimum"=w382:dbl)  [unwired: 2 in, 2 out]
            n133 = Unbundle By Name(w387) -> ("m/z"=w372:dbl[])
            n134 = Index Array(array=w386) -> (element=w373:cluster{dbl[], "Amplitudes":dbl[]})  [unwired: 1 in]
            n135 = Array Max & Min(array=w372) -> (max value=w388:dbl)  [unwired: 3 out]
            n136 = Unbundle(w373) -> (w385:dbl[], "Amplitudes"=w384:dbl[])
            n137 = for {
              tunnel: w384 -> [w391] mode=indexing
              tunnel: w385 -> [w395] mode=indexing
              tunnel: w382 -> [w394]
              tunnel: w383 -> [w393]
              tunnel: [w390] -> w374 mode=indexing
              n138 = In Range and Coerce(upper limit=w393, x=w395, lower limit=w394) -> (In Range?=w392:bool)  [unwired: 1 out]
              n139 = case shown="True" w392 {
                tunnel: w391 -> [_ w396]
                tunnel: [_ w396] -> w390
                frame False {
                  (unwired) nan
                }
                frame True {
                }
              }
            }
            n140 = Array Max & Min(array=w374) -> (max value=w376:dbl, min value=w375:dbl)  [unwired: 2 out]
            n141 = property on="Spectrum" class="XYGraph (strict)"("XScale.Minimum"=0.0 ("X Scale.Range:Minimum"), "XScale.Maximum"=w388) -> ()  [unwired: 2 in, 2 out]
            n142 = Subtract(x=w376, y=w375) -> (x-y=w379:dbl)
            n143 = Multiply(x=w379, y=0.05) -> (x*y=w377:dbl)
            n144 = Add(x=w376, y=w377) -> (x+y=w381:dbl)
            n145 = Subtract(x=w375, y=w377) -> (x-y=w380:dbl)
            n146 = property on="Spectrum" class="XYGraph (strict)"("YScale.Maximum"=w381, "YScale.Minimum"=w380) -> ()  [unwired: 2 in, 2 out]
          }
        }
      }
      event "Add to": Value Change {
        n147 = event-data() -> ()  [unwired: 1 in, 1 out]
        n148 = Unbundle By Name(w404) -> ("Peaks Table"=w405:dbl[][])
        n149 = local read "Original m/z"() -> (w400:dbl)
        n150 = Build Array(w400, "time", "m/z") -> (w398:dbl[])
        n151 = Build Array (concatenate)(w405, w398) -> (w399:dbl[][])
        n152 = local write "Tab Control"(T2."Assigned Peaks" ("Tab Control")) -> ()
        n153 = Bundle By Name(cluster=w404, "Peaks Table"=w399) -> (w403:T7)
      }
      event "Spectrum": Scale Range Change; "Binning", "BinWidth", "Res.": Value Change {
        n154 = event-data() -> ()  [unwired: 1 in, 1 out]
      }
      event "Calc Calibration": Value Change {
        w426 = "\n"
        w454 = 100
        w459 = T10 0 items=["Least Square", "Least Absolute Residual", "Bisquare"] ("method")
        w460 = T11 0 items=["SVD", "Givens", "Givens2", "Householder", "LU Decomposition", "Cholesky", "SVD for Rank Deficient H"] ("algorithm")
        n155 = event-data() -> ()  [unwired: 1 in, 1 out]
        n156 = Unbundle By Name(w440) -> ("BinnedSpec.Intensity"=w439:dbl[], "Spectrum.TrigDelay"=w419:dbl, "Spectrum.SampleRate"=w420:dbl)
        n157 = Index Array(array="Calibration Table", index (col) #1=1 ("disabled index (col)"), index (col) #2=2 ("index (col)")) -> (element #1=w418:dbl[], element #2=w411:dbl[])  [unwired: 2 in]
        n158 = Index Array(array="Calibration Table", index (col)=2 ("disabled index (col)")) -> (element=w434:dbl[])  [unwired: 1 in]
        n159 = Divide(x=1000000.0, y=w420) -> (x/y=w421:dbl)
        n160 = Array Size(array=w439) -> (size(s)=w438:i32)
        n161 = Multiply(x=w419, y=w421) -> (x*y=w422:dbl)
        n162 = call <vilib>:"General Polynomial Fit.vi"("Y"=w411, "polynomial order"=2, "X"=w418, "method"=w459, "algorithm"=w460) -> ("Best Polynomial Fit"=w410:dbl[], "Polynomial Coefficients"=w452:dbl[])  [unwired: 7 in, 2 out]
        n163 = Array Max & Min(array=w418) -> (max value=w457:dbl, min value=w456:dbl)  [unwired: 2 out]
        n164 = Subtract(x=w410, y=w434) -> (x-y=w433:dbl[])
        n165 = for {
          N: w438 -> [_]
          shift-right: [w462] -> _
          shift-left: w422 -> [w463]
          tunnel: [w462] -> w442 mode=indexing
          tunnel: w421 -> [w461]
          n166 = Add(x=w463, y=w461) -> (x+y=w462:dbl)
        }
        n167 = Subtract(x=w457, y=w456) -> (x-y=w455:dbl)
        n168 = Index Array(array=w452) -> (element #1=w449:dbl, element #2=w450:dbl, element #3=w451:dbl)  [unwired: 3 in]
        n169 = Insert Into Array(array="Calibration Table", index (col)=3 ("disabled index (col)"), new element=w433) -> (w431:dbl[][])  [unwired: 1 in]
        n170 = Divide(x=w455, y=w454) -> (x/y=w453:dbl)
        n171 = Reverse 1D Array(array=w452) -> (reversed array=w412:dbl[])
        n172 = for {
          N: w454 -> [_]
          tunnel: w456 -> [w472]
          tunnel: w453 -> [w475]
          tunnel: w451 -> [w470]
          tunnel: w450 -> [w469]
          tunnel: w449 -> [w466]
          tunnel: [w465] -> w414 mode=indexing
          tunnel: [w464] -> w415 mode=indexing
          i -> [w474]
          n173 = Multiply(x=w475, y=w474) -> (x*y=w473:dbl)
          n174 = Add(x=w472, y=w473) -> (x+y=w464:dbl)
          n175 = Square(x=w464) -> (x^2=w471:dbl)
          n176 = Multiply(x=w470, y=w471) -> (x*y=w467:dbl)
          n177 = Multiply(x=w469, y=w464) -> (x*y=w468:dbl)
          n178 = Compound Arithmetic op=ADD(w466, w468, w467) -> (w465:dbl)
        }
        n179 = local write "Calibration Coefficients"(w412) -> ()
        n180 = Index Array(array=w412) -> (element #1=w443:dbl, element #2=w444:dbl, element #3=w445:dbl)  [unwired: 3 in]
        n181 = Compound Arithmetic op=MULTIPLY(w442, w442, w443) -> (w447:dbl[])
        n182 = Compound Arithmetic op=MULTIPLY(w444, w442) -> (w446:dbl[])
        n183 = Compound Arithmetic op=ADD(w447, w446, w445) -> (w424:dbl[])
        n184 = local write "Tab Control"(T2."Results" ("Tab Control")) -> ()
        n185 = Array To Spreadsheet String(delimiter (Tab)=w426, array=w424, 3:"%f" ("format string")) -> (spreadsheet string=w427:string)
        n186 = Bundle("Calibration Table"=w418, "Calibration Table"=w411) -> (w417:T12)  [unwired: 1 in]
        n187 = Bundle(w415, w414) -> (w416:cluster{dbl[], dbl[]})  [unwired: 1 in]
        n188 = Build Array(w417, w416) -> (→"M/z curve fitting":T13)
        n189 = call <vilib>:"Goodness of Fit.vi"("Best Fit"=w410, "Y"=w411) -> ("R-square"=→"R^2":dbl)  [unwired: 6 in, 3 out]
        n190 = Concatenate Strings("m/z" ("string"), w426, w427) -> (w428:string)
        n191 = Bundle By Name(cluster=w440, "m/z"=w424, "Peaks Table"=w431, "Spectrum.Calibr."=w412) -> (w448:T7)
        n192 = invoke class="App" method="Clipboard.Write"("Param 0"=w428) -> ()  [unwired: 3 in, 4 out]
      }
      event "Apply": Value Change {
        w486 = "\n"
        n193 = event-data() -> ()  [unwired: 1 in, 1 out]
        n194 = Unbundle By Name(w482) -> ("BinnedSpec.Intensity"=w491:dbl[], "Spectrum.TrigDelay"=w477:dbl, "Spectrum.SampleRate"=w478:dbl)
        n195 = Divide(x=1000000.0, y=w478) -> (x/y=w480:dbl)
        n196 = Array Size(array=w491) -> (size(s)=w490:i32)
        n197 = Multiply(x=w477, y=w480) -> (x*y=w481:dbl)
        n198 = for {
          N: w490 -> [_]
          shift-right: [w500] -> _
          shift-left: w481 -> [w501]
          tunnel: [w500] -> w493 mode=indexing
          tunnel: w480 -> [w499]
          n199 = Add(x=w501, y=w499) -> (x+y=w500:dbl)
        }
        n200 = Index Array(array="Calibration Coefficients") -> (element #1=w494:dbl, element #2=w495:dbl, element #3=w496:dbl)  [unwired: 3 in]
        n201 = Compound Arithmetic op=MULTIPLY(w493, w493, w494) -> (w498:dbl[])
        n202 = Compound Arithmetic op=MULTIPLY(w495, w493) -> (w497:dbl[])
        n203 = Compound Arithmetic op=ADD(w498, w497, w496) -> (w484:dbl[])
        n204 = Array To Spreadsheet String(delimiter (Tab)=w486, array=w484, 3:"%f" ("format string")) -> (spreadsheet string=w487:string)
        n205 = Concatenate Strings("m/z" ("string"), w486, w487) -> (w488:string)
        n206 = Bundle By Name(cluster=w482, "m/z"=w484, "Spectrum.Calibr."="Calibration Coefficients") -> (w483:T7)
        n207 = invoke class="App" method="Clipboard.Write"("Param 0"=w488) -> ()  [unwired: 3 in, 4 out]
      }
      event "Export_GraphData": Value Change {
        w505 = "\t"
        n208 = event-data() -> ()  [unwired: 1 in, 1 out]
        n209 = control-ref of="Spectrum"() -> (w518:refnum<vi>)
        n210 = property class="XYGraph (strict)"(reference=w518) -> ("Value"=w517:cluster{dbl[], "Amplitudes":dbl[]}[])  [unwired: 1 in, 2 out]
        n211 = Index Array(array=w517) -> (element=w516:cluster{dbl[], "Amplitudes":dbl[]})  [unwired: 1 in]
        n212 = Unbundle(w516) -> (w513:dbl[], "Amplitudes"=w515:dbl[])
        n213 = Array Size(array=w513) -> (size(s)=w512:i32)
        n214 = Build Array(w513, w515) -> (w514:dbl[][])
        n215 = Transpose 2D Array(2D array=w514) -> (transposed array=w510:dbl[][])
        n216 = Subtract(x=w512, y=2) -> (x-y=w508:i32)
        n217 = Array Subset(array=w510, index (row)=1 ("index"), length (row)=w508) -> (w507:dbl[][])  [unwired: 2 in]
        n218 = Unbundle By Name(w503) -> ("Filename"=w502:string)
        n219 = Array To Spreadsheet String(delimiter (Tab)=w505, array=w507, 3:"%_6g" ("format string")) -> (spreadsheet string=w520:string)
        n220 = Concatenate Strings("m/z" ("string"), w505, w502, "\r", w520) -> (w521:string)
        n221 = invoke class="App" method="Clipboard.Write"("Param 0"=w521) -> ()  [unwired: 3 in, 4 out]
      }
      event "ApplyToFile": Value Change {
        n222 = event-data() -> ()  [unwired: 1 in, 1 out]
        n223 = Unbundle By Name(w534) -> ("InitialCali."=w532:dbl[], "Spectrum"=w533:T5)
        n224 = control-ref of="Path"() -> (w531:refnum<vi>)
        n225 = property class="Path"(reference=w531) -> ("Value"=w526:path)  [unwired: 1 in, 2 out]
        n226 = Path To String(path=w526) -> (string=w529:string)
        n227 = Concatenate Strings(w529, ".bak" ("string")) -> (w528:string)
        n228 = String To Path(string=w528) -> (path=w527:path)
        n229 = Move(source path=w526, 9:TRUE ("overwrite (F)"), 10:w527) -> (error out=w524:errorcluster)  [unwired: 2 in, 2 out]
        n230 = call "WriteTextFile.vi"("overwrite? (F)"=TRUE ("Overwrite?"), "InitialCali."=w532, "error in (no error)"=w524, "Signal Segment"=w533, "Filename"=w526) -> ()  [unwired: 6 in, 1 out]
      }
      event "ApplyToMainProgram": Value Change {
        n231 = event-data() -> ()  [unwired: 1 in, 1 out]
        n232 = Unbundle By Name(w537) -> ("Spectrum.Calibr."=w536:dbl[])
        n233 = property class="Arr (strict)"(reference=w535, "Val(Sgnl)"=w536) -> ()  [unwired: 1 in, 2 out]
      }
      event "mzML Export": Value Change {
        n234 = event-data() -> ()  [unwired: 1 in, 1 out]
        n235 = Unbundle By Name(w547) -> ("Spectrum"=w545:T5)  [unwired: 1 out]
        n236 = control-ref of="Path"() -> (w546:refnum<vi>)
        n237 = property class="Path"(reference=w546) -> ("Value"=w544:path)  [unwired: 1 in, 2 out]
        n238 = Strip Path(path=w544) -> (stripped path=w543:path, name=w542:string)
        n239 = xnode "Match Regular Expression"("input string"=w542, "regular expression"="(.[0-9a-zA-Z~]+$)") -> ("before match"=w541:string, "error out"=w538:errorcluster)  [unwired: 4 in, 4 out]
        n240 = Build Path(base path=w543, name or relative path=w541) -> (appended path=w539:path)
        n241 = call "Write_mzMLFile.vi"("error in (no error)"=w538, "Signal Segment"=w545, "Filename"=w539) -> ()  [unwired: 8 in, 1 out]
      }
      event "Search": Value Change {
        n242 = event-data() -> ()  [unwired: 1 in, 1 out]
        n243 = call <vilib>:"Set Busy.vi"() -> ("error out"=w661:errorcluster)  [unwired: 10 in, 1 out]
        n244 = flat-sequence {
          tunnel: w666 -> [w680]
          tunnel: [w679] -> w664
          tunnel: [w667] -> w662
          tunnel: w661 -> [w667]
          frame #0 {
            n245 = Unbundle By Name(w680) -> ("BinnedSpec.m/z"=w678:dbl[], "BinnedSpec.Intensity"=w677:dbl[])
            n246 = call <vilib>:"Peak Detector.vi"("peaks/valleys"=enum32{"Peaks", "Valleys"}."Peaks", "width"="width", "threshold"="threshold", "X"=w677) -> ("Amplitudes"=w670:dbl[], "Locations"=w681:dbl[], "# found"=→"# found":i32)  [unwired: 3 in, 2 out]
            n247 = control-ref of="Multicolumn Listbox"() -> (w672:refnum<vi>)
            n248 = for {
              tunnel: w678 -> [w691]
              tunnel: w681 -> [w690] mode=indexing
              tunnel: [w689] -> w671 mode=indexing
              n249 = Interpolate 1D Array(1:w690, 2:w691) -> (0:w689:dbl)
            }
            n250 = Bundle(w671, "Amplitudes"=w670) -> (w679:cluster{dbl[], "Amplitudes":dbl[]})  [unwired: 1 in]
            n251 = for {
              tunnel: w671 -> [w687] mode=indexing
              tunnel: w670 -> [w686] mode=indexing
              tunnel: [w683] -> w669 mode=indexing
              n252 = Format Value(format string="%1.2f", value (0)=w687) -> (output string=w685:string)  [unwired: 1 in]
              n253 = Format Value(format string="%1.7f", value (0)=w686) -> (output string=w684:string)  [unwired: 1 in]
              n254 = Build Array(w685, w684) -> (w683:string[])
            }
            n255 = property class="MCListbox (strict)"(reference=w672, "ItemNames"=w669, "ColHdrString"=string[] ["m/z", "Intensity"]) -> ()  [unwired: 1 in, 2 out]
          }
        }
        n256 = call <vilib>:"Unset Busy.vi"("error in (no error)"=w662) -> ()  [unwired: 10 in, 1 out]
        n257 = Bundle By Name(cluster=w666, "PeaksList"=w664) -> (w665:T7)
      }
      event "ExportPCA": Value Change {
        n258 = event-data() -> ()  [unwired: 1 in, 1 out]
        n259 = call <vilib>:"Set Busy.vi"() -> ("error out"=w693:errorcluster)  [unwired: 10 in, 1 out]
        n260 = flat-sequence {
          tunnel: w696 -> [w708]
          tunnel: [w699] -> w694
          tunnel: [w697] -> w692
          tunnel: w693 -> [w697]
          frame #0 {
            w704 = 750 ("dimension size")
            n261 = for {
              N: w704 -> [_]
              shift-right: [w710] -> _
              shift-left: 50.0 -> [w709]
              tunnel: [w709] -> w700 mode=indexing
              n262 = Increment(x=w709) -> (x+1=w710:dbl)
            }
            n263 = Initialize Array(0.0 ("element"), w704) -> (w705:dbl[])
            n264 = Unbundle By Name(w708) -> ("PeaksList.m/z"=w703:dbl[], "PeaksList.Intensity"=w702:dbl[])
            n265 = for {
              N: w704 -> [_]
              shift-right: [w730] -> w701
              shift-left: w705 -> [w731]
              tunnel: w700 -> [w729]
              tunnel: w703 -> [w728] mode=indexing
              tunnel: w702 -> [w726] mode=indexing
              shift-right: [w720] -> _
              shift-left: 0.0 -> [w727]
              shift-right: [w719] -> _
              shift-left: _ -> [w718]
              i -> [w724]
              # "tracking last 10 peaks offset"
              n266 = Equal To 0?(x=w724) -> (x = 0?=w725:bool)
              n267 = Threshold 1D Array(1:w727, 2:w728, 3:w729) -> (0:w720:dbl)
              n268 = Round To Nearest(number=w720) -> (nearest integer value=w721:dbl)
              n269 = Subtract(x=w720, y=w721) -> (x-y=w713:dbl)
              n270 = Round Toward -Infinity(1:w720) -> ()  [unwired: 1 out]
              n271 = To Long Integer(number=w721) -> (32bit integer=w715:i32)
              n272 = call <vilib>:"Mean PtByPt.vi"("x"=w713, "sample length"=10, "initialize"=w725) -> ("mean"=w719:dbl)  [unwired: 1 in, 1 out]
              n273 = Sign(1:w718) -> (0:w717:dbl)
              n274 = Sign(1:w713) -> (0:w712:dbl)
              n275 = Add(x=w715, y=w712) -> (x+y=w716:dbl)
              n276 = Equal?(x=w712, y=w717) -> ()  [unwired: 1 out]
              n277 = To Long Integer(number=w716) -> (32bit integer=w714:i32)
              n278 = Select(t=w715, s=TRUE, f=w714) -> (s? t:f=w722:i32)
              n279 = in-place {
                in-place-border: w726 -> [w732]
                n280 = in-place-array #1(w731, w722) -> ()  [unwired: 1 out]
                n281 = in-place-array #1(w732) -> (w730:dbl[])  [unwired: 1 out]
              }
            }
            n282 = Bundle(w700, w701) -> (w699:cluster{dbl[], dbl[]})  [unwired: 1 in]
          }
        }
        n283 = Bundle By Name(cluster=w696, "PCA"=w694) -> (w695:T7)
        n284 = call <vilib>:"Unset Busy.vi"("error in (no error)"=w692) -> ()  [unwired: 10 in, 1 out]
      }
      event "AddSelection": Value Change {
        n285 = event-data() -> ()  [unwired: 1 in, 1 out]
        n286 = control-ref of="Multicolumn Listbox"() -> (w737:refnum<vi>)
        n287 = property class="MCListbox (strict)"(reference=w737) -> (reference out=w736:refnum<vi>, error out=w735:errorcluster, "Value"=w733:i32[])  [unwired: 1 in]
        n288 = property class="MCListbox (strict)"(reference=w736, error in=w735) -> ("ItemNames"=w734:string[][])  [unwired: 2 out]
        n289 = for {
          tunnel: w734 -> [w740] mode=indexing
          tunnel: w733 -> [w739] mode=indexing
          n290 = Array Subset(array=w740, index=w739) -> ()  [unwired: 1 in, 1 out]
        }
      }
      event "Calibration Table": Value Change {
        n291 = event-data() -> ()  [unwired: 1 in, 1 out]
        n292 = local read "Calibration Table"() -> (w741:dbl[][])
        n293 = Bundle By Name(cluster=w743, "Peaks Table"=w741) -> (w742:T7)
      }
      event "Selected Peak list": Edit Cell? {
        n294 = event-data() -> ("String"=w746:string)  [unwired: 1 in]
        n295 = xnode "Match Regular Expression"("input string"=w746, "regular expression"="([-+]?[0-9]*\\.?[0-9]+)([eE][-+]?[0-9]+)?") -> ("whole match"=w744:string)  [unwired: 4 in, 4 out]
        n296 = event-data("String"=w744) -> ()  [unwired: 2 in, 1 out]
      }
      event "CalcPeakAreas": Value Change {
        n297 = event-data() -> ()  [unwired: 1 in, 1 out]
        n298 = control-ref of="Selected Peak list"() -> (w874:refnum<vi>)
        n299 = Unbundle By Name(w872) -> ("m/z"=w867:dbl[], "Spectrum.Spectrum"=w861:sgl[])
        n300 = property class="MCListbox (strict)"(reference=w874) -> (reference out=w873:refnum<vi>, "ItemNames"=w864:string[][])  [unwired: 1 in, 1 out]
        n301 = control-ref of="CalcPeakAreas"() -> (w860:refnum<vi>)
        n302 = Index Array(array=w864, index (col) #1=0 ("disabled index (col)"), index (col) #2=1 ("index (col)")) -> (element #1=w871:string[], element #2=w868:string[])  [unwired: 2 in]
        n303 = property class="Bool (strict)"(reference=w860, "Value"=FALSE) -> ()  [unwired: 1 in, 2 out]
        n304 = for {
          tunnel: w871 -> [w891] mode=indexing
          tunnel: w868 -> [w890] mode=indexing
          tunnel: [w883] -> w866 mode=indexing if=w884
          tunnel: [w888] -> w865 mode=indexing if=w884
          w887 = nan ("default (0 DBL)")
          n305 = Fract/Exp String To Number(string=w891, default (0 dbl)=w887) -> (number=w885:dbl)  [unwired: 2 in, 1 out]
          n306 = Fract/Exp String To Number(string=w890, default (0 dbl)=w887) -> (number=w889:dbl)  [unwired: 2 in, 1 out]
          n307 = Subtract(x=w885, y=w889) -> (x-y=w883:dbl)
          n308 = Add(x=w885, y=w889) -> (x+y=w888:dbl)
          n309 = Not A Number/Path/Refnum?(number/path/refnum=w883) -> (NaN/Path/Refnum?=w886:bool)
          n310 = Not(x=w886) -> (.not. x?=w884:bool)
        }
        n311 = call "CalcPeakArea.vi"("spectrum"=w861, "m/z in"=w867, "to"=w865, "from"=w866) -> ("Peak Area"=w862:dbl[])  [unwired: 7 in]
        n312 = for {
          tunnel: w862 -> [w876] mode=indexing
          shift-right: [w877] -> w863
          shift-left: w864 -> [w879]
          i -> [w875]
          n313 = in-place {
            in-place-border: w876 -> [w880]
            n314 = in-place-array #2(w879, w875, 2) -> ()  [unwired: 1 out]
            n315 = Format Into String(format string="%_4g", w880) -> (resulting string=w881:string)  [unwired: 2 in, 1 out]
            n316 = in-place-array #2(w881) -> (w877:string[][])  [unwired: 2 out]
          }
        }
        n317 = property class="MCListbox (strict)"(reference=w873, "ItemNames"=w863) -> ()  [unwired: 1 in, 2 out]
      }
      event "CopyPeakAreas": Value Change {
        w895 = "\n"
        n318 = event-data() -> ()  [unwired: 1 in, 1 out]
        n319 = control-ref of="Selected Peak list"() -> (w902:refnum<vi>)
        n320 = property class="MCListbox (strict)"(reference=w902) -> ("ItemNames"=w900:string[][])  [unwired: 1 in, 2 out]
        n321 = Index Array(array=w900, index (col)=2 ("disabled index (col)")) -> (element=w899:string[])  [unwired: 1 in]
        n322 = for {
          tunnel: w899 -> [w907] mode=indexing
          tunnel: [w903] -> w894 mode=indexing if=w904
          n323 = Fract/Exp String To Number(string=w907, default (0 dbl)=nan ("default (0 DBL)")) -> (number=w903:dbl)  [unwired: 2 in, 1 out]
          n324 = Not A Number/Path/Refnum?(number/path/refnum=w903) -> (NaN/Path/Refnum?=w905:bool)
          n325 = Not(x=w905) -> (.not. x?=w904:bool)
        }
        n326 = Unbundle By Name(w893) -> ("Filename"=w892:string)
        n327 = Array To Spreadsheet String(delimiter (Tab)=w895, array=w894, 3:"%_4g" ("format string")) -> (spreadsheet string=w896:string)
        n328 = Concatenate Strings(w892, w895, w896) -> (w897:string)
        n329 = invoke class="App" method="Clipboard.Write"("Param 0"=w897) -> ()  [unwired: 3 in, 4 out]
      }
      event "ExportTable": Value Change {
        n330 = event-data() -> ()  [unwired: 1 in, 1 out]
        n331 = Unbundle By Name(w915) -> ("AccumulatedPeakAreas.Labels"=w908:string[], "AccumulatedPeakAreas.Areas"=w911:dbl[][])
        n332 = disable-structure "Diagram Disable Structure" shown="Enabled" {
          disable-tunnel: w911 -> [w921 w927]
          disable-tunnel: [w920 w927] -> w910
          disable-tunnel: [w919 w926] -> w909
          disable-tunnel: w908 -> [w919 w926]
          frame Disabled {
            # "Ratio calculation"
            n333 = for {
              tunnel: w921 -> [w925] mode=indexing
              tunnel: [w922] -> w920 mode=indexing
              n334 = Index Array(array=w925, index=0) -> (element=w924:dbl)
              n335 = Divide(x=w925, y=w924) -> (x/y=w922:dbl[])
            }
          }
          frame Enabled {
            # "Direct output"
          }
        }
        n336 = Transpose 2D Array(2D array=w910) -> (transposed array=w914:dbl[][])
        n337 = Array To Spreadsheet String(array=w909, 3:"%s" ("format string")) -> (spreadsheet string=w913:string)  [unwired: 1 in]
        n338 = Array To Spreadsheet String(array=w914, 3:"%_4g" ("format string")) -> (spreadsheet string=w916:string)  [unwired: 1 in]
        n339 = Concatenate Strings(w913, w916) -> (w917:string)
        n340 = invoke class="App" method="Clipboard.Write"("Param 0"=w917) -> ()  [unwired: 3 in, 4 out]
      }
      event "Export+Proc": Value Change {
        n341 = event-data() -> ()  [unwired: 1 in, 1 out]
        n342 = Unbundle By Name(w933) -> ("AccumulatedPeakAreas.Labels"=w932:string[], "AccumulatedPeakAreas.Areas"=w928:dbl[][], "AccumulatedPeakAreas.Areas^2"=w931:dbl[][], "AccumulatedPeakAreas.n"=w930:i32[])
        n343 = disable-structure "Diagram Disable Structure" shown="Enabled" {
          disable-tunnel: w928 -> [w937 w945]
          disable-tunnel: w932 -> [w939 w946]
          disable-tunnel: w931 -> [w936 _]
          disable-tunnel: w930 -> [w935 _]
          disable-tunnel: [w938 w944] -> w929
          frame Enabled {
            # "Need to test the validaty of this part"
            # "ratio calculation"
            n344 = call "GetStatistics_Array.vi"("n"=w935, "sum_X^2"=w936, "sum_X"=w937) -> ("Table"=w934:dbl[][])  [unwired: 8 in]
            n345 = Array To Spreadsheet String(array=w934, 3:"%_4g" ("format string")) -> (spreadsheet string=w941:string)  [unwired: 1 in]
            n346 = Array To Spreadsheet String(array=w939, 3:"%s\\t" ("format string")) -> (spreadsheet string=w942:string)  [unwired: 1 in]
            n347 = Concatenate Strings(w942, w941) -> (w938:string)
          }
          frame Disabled {
            # "Direct output"
            n348 = Transpose 2D Array(2D array=w945) -> (transposed array=w949:dbl[][])
            n349 = Array To Spreadsheet String(array=w946, 3:"%s" ("format string")) -> (spreadsheet string=w950:string)  [unwired: 1 in]
            n350 = Array To Spreadsheet String(array=w949, 3:"%_4g" ("format string")) -> (spreadsheet string=w948:string)  [unwired: 1 in]
            n351 = Concatenate Strings(w950, w948) -> (w944:string)
          }
        }
        n352 = invoke class="App" method="Clipboard.Write"("Param 0"=w929) -> ()  [unwired: 3 in, 4 out]
      }
      event "Accumulate": Value Change {
        n353 = event-data() -> ()  [unwired: 1 in, 1 out]
        n354 = property class="MCListbox (strict)"(reference=w963) -> ("ItemNames"=w969:string[][])  [unwired: 1 in, 2 out]
        n355 = Unbundle By Name(w967) -> ("Filename"=w961:string, "AccumulatedPeakAreas.Labels"=w962:string[], "AccumulatedPeakAreas.Areas"=w960:dbl[][], "AccumulatedPeakAreas.Areas^2"=w959:dbl[][], "AccumulatedPeakAreas.n"=w957:i32[])
        n356 = Search 1D Array(1D array=w962, element=w961) -> (index of element=w954:i32)  [unwired: 1 in]
        n357 = Index Array(array=w969, index (col)=2 ("disabled index (col)")) -> (element=w968:string[])  [unwired: 1 in]
        n358 = for {
          tunnel: w968 -> [w1004] mode=indexing
          tunnel: [w1000] -> w958 mode=indexing if=w1001
          n359 = Fract/Exp String To Number(string=w1004, default (0 dbl)=nan ("default (0 DBL)")) -> (number=w1000:dbl)  [unwired: 2 in, 1 out]
          n360 = Not A Number/Path/Refnum?(number/path/refnum=w1000) -> (NaN/Path/Refnum?=w1002:bool)
          n361 = Not(x=w1002) -> (.not. x?=w1001:bool)
        }
        n362 = case shown="0.." w954 {
          selector: w954 -> [w971 _]
          tunnel: [w987 w999] -> w965
          tunnel: w962 -> [w987 w998]
          tunnel: w961 -> [w972 w988]
          tunnel: w960 -> [w985 w997]
          tunnel: w959 -> [w976 w996]
          tunnel: w958 -> [w979 w995]
          tunnel: w957 -> [w973 w993]
          tunnel: [w986 w991] -> w952
          tunnel: [w975 w990] -> w956
          tunnel: [w974 w989] -> w955
          tunnel: [w972 w988] -> w953
          frame 0.. {
            n363 = Index Array(array=w985, index (row)=w971) -> (element=w984:dbl[])  [unwired: 1 in]
            n364 = Index Array(array=w976, index (row)=w971) -> (element=w982:dbl[])  [unwired: 1 in]
            n365 = Index Array(array=w973, index=w971) -> (element=w980:i32)
            n366 = Square(x=w979) -> (x^2=w978:dbl[])
            n367 = Add(x=w984, y=w979) -> (x+y=w983:dbl[])
            n368 = Add(x=w982, y=w978) -> (x+y=w977:dbl[])
            n369 = Increment(x=w980) -> (x+1=w981:i32)
            n370 = Replace Array Subset(array=w985, new element=w983, index (row)=w971) -> (w986:dbl[][])  [unwired: 1 in]
            n371 = Replace Array Subset(array=w976, new element=w977, index (row)=w971) -> (w975:dbl[][])  [unwired: 1 in]
            n372 = Replace Array Subset(array=w973, new element=w981, index=w971) -> (w974:i32[])
          }
          frame -1, Default {
            n373 = Square(x=w995) -> (x^2=w994:dbl[])
            n374 = Build Array (concatenate)(w998, w988) -> (w999:string[])
            n375 = Build Array (concatenate)(w997, w995) -> (w991:dbl[][])
            n376 = Build Array (concatenate)(w996, w994) -> (w990:dbl[][])
            n377 = Build Array (concatenate)(w993, 1 ("element")) -> (w989:i32[])
          }
        }
        "Accumulated Data" <- w952
        n378 = Enqueue Element(queue=w964, element=w953) -> ()  [unwired: 2 in, 3 out]
        n379 = Bundle By Name(cluster=w967, "AccumulatedPeakAreas.Labels"=w965, "AccumulatedPeakAreas.Areas"=w952, "AccumulatedPeakAreas.Areas^2"=w956, "AccumulatedPeakAreas.n"=w955) -> (w966:T7)
      }
      event "Reset": Value Change {
        n380 = event-data() -> ()  [unwired: 1 in, 1 out]
        n381 = Bundle By Name(cluster=w1008, "AccumulatedPeakAreas"=T8 {"Labels"=[], "Areas"=[], "Areas^2"=[], "n"=[]}) -> (w1007:T7)
        n382 = Unbundle By Name(w1007) -> ("AccumulatedPeakAreas.Areas"=w1006:dbl[][])
        n383 = property on="Accumulated Data" class="Arr (strict)"("Value"=w1006) -> ()  [unwired: 2 in, 2 out]
      }
    }
    n384 = Unbundle By Name(w37) -> ("Peaks Table"=w42:dbl[][], "m/z"=w40:dbl[], "Spectrum.Spectrum"=w39:sgl[], "PeaksList"=w35:cluster{"m/z":dbl[], "Intensity":dbl[]}, "PCA"=w34:cluster{"m/z":dbl[], "Intensity":dbl[]})
    n385 = control-ref of="Spectrum"() -> (w33:refnum<vi>)
    n386 = local write "Calibration Table"(w42) -> ()
    n387 = case shown="True" w38 {
      tunnel: w40 -> [_ w59]
      tunnel: w39 -> [_ w58]
      tunnel: w33 -> [_ w46]
      tunnel: w37 -> [w44 w51]
      tunnel: [w44 w50] -> w36
      tunnel: w35 -> [_ w48]
      tunnel: w34 -> [_ w47]
      frame False {
      }
      frame True {
        n388 = call <vilib>:"Set Busy.vi"("disable click? (T)"=FALSE) -> ("error out"=w54:errorcluster)  [unwired: 9 in, 1 out]
        n389 = call-poly "SpecBinning.vi"("BinType"="BinType", "BinWidth"="BinWidth", "Binning"="Binning", "error in (no error)"=w54, "Signal"=w58, "m/z Array"=w59, "GraphsRef."=w46) -> ("error out"=w53:errorcluster, "BinnedSpectrum"=w45:cluster{"m/z Array":dbl[], "Signal":dbl[]})  [unwired: 3 in]
        n390 = call <vilib>:"Unset Busy.vi"("error in (no error)"=w53) -> ()  [unwired: 10 in, 1 out]
        n391 = Build Array(w45, w48, w47) -> (w49:cluster{"m/z":dbl[], "Intensity":dbl[]}[])
        n392 = disable-structure shown="Enabled" {
          disable-tunnel: w46 -> [w62 _]
          disable-tunnel: w45 -> [w61 _]
          frame Enabled {
            n393 = call-poly "FindMassResolution.vi"("EnableResDisplay"="Res.", "BinnedSpectrum"=w61, "GraphRef."=w62) -> ()  [unwired: 7 in, 2 out]
          }
          frame Disabled {
          }
        }
        n394 = property class="XYGraph (strict)"(reference=w46, "Value"=w49) -> ()  [unwired: 1 in, 2 out]
        n395 = Bundle By Name(cluster=w51, "BinnedSpec"=w45) -> (w50:T7)
      }
    }
  }
  "Referance Mass" <- string[][] [["Compound", "", "m/z", ""], ["Sexithiophene", "6T", "493.9420", "s"], ["", "4T", "329.9665", "s"], ["", "5T-2H", "407.9230", ""], ["", "8T", "657.9174", "w"], ["C60", "M+", "720.0000", ""], ["NPM", "M+", "297.0890", "s"], ["CHCA", "M+", "189.04", "s"], ["DHB", "M+", "154.03", "s"]] ("Referance Mass")
